vi "Tractor.vi"(1 "Y":dbl, 2 "X":dbl) -> (0 "XY Graph":cluster{dbl[], dbl[]}(graph))   [LabVIEW 2022 SP3]
panel:
  out "Array":dbl[](array[numeric])
  out "appended array":dbl[](array[numeric])
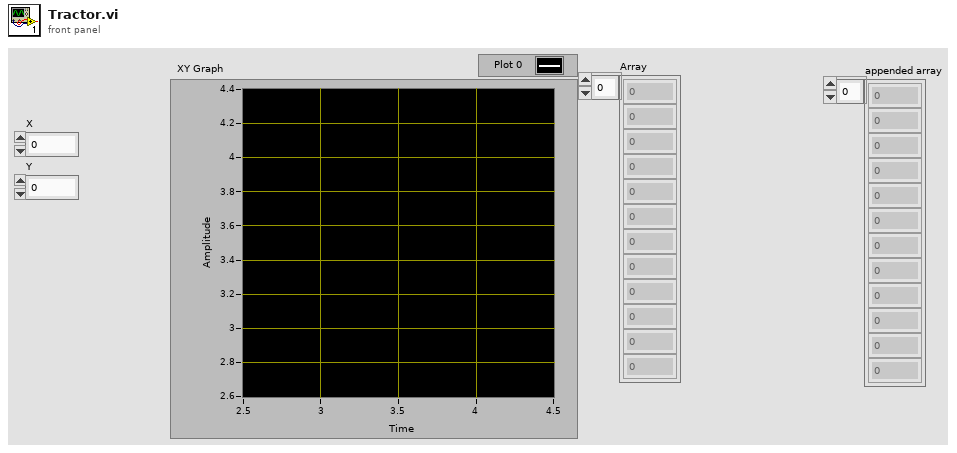
[diagram p1: front panel]
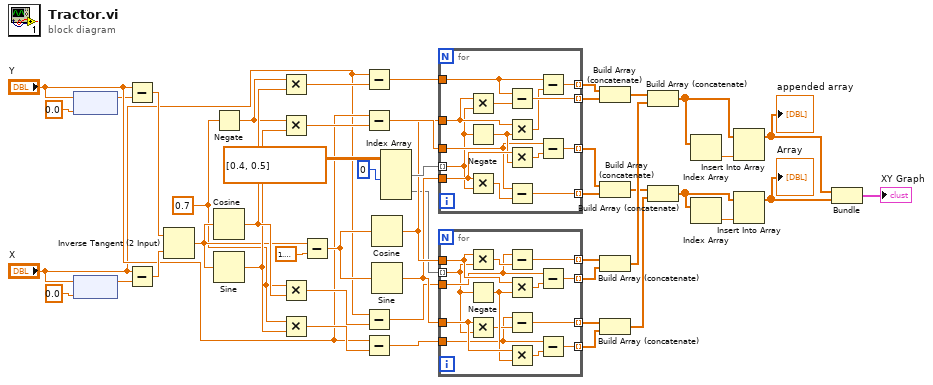
[diagram p0: block diagram]
diagram:
  w2 = 0.7 ("x")
  n1 = feedback #1(0.0 ("Y")) -> (w6:dbl)
  n2 = feedback-in #1("Y") -> ()
  n3 = feedback #2(0.0 ("Y")) -> (w3:dbl)
  n4 = feedback-in #2("X") -> ()
  n5 = Subtract(x="Y", y=w6) -> (x-y=w48:dbl)
  n6 = Subtract(x="X", y=w3) -> (x-y=w47:dbl)
  n7 = Inverse Tangent (2 Input)(1:w47, 2:w48) -> (0:w12:dbl)
  n8 = Negate(x=w2) -> (-x=w1:dbl)
  n9 = Cosine(x=w12) -> (cos(x)=w30:dbl)
  n10 = Sine(x=w12) -> (sin(x)=w29:dbl)
  n11 = Multiply(x=w1, y=w30) -> (x*y=w31:dbl)
  n12 = Multiply(x=w1, y=w29) -> (x*y=w44:dbl)
  n13 = Multiply(x=w2, y=w30) -> (x*y=w27:dbl)
  n14 = Multiply(x=w2, y=w29) -> (x*y=w26:dbl)
  n15 = Subtract(x=w12, y=1.5707963267948966) -> (x-y=w39:dbl)
  n16 = Subtract(x="X", y=w31) -> (x-y=w32:dbl)
  n17 = Subtract(x="Y", y=w44) -> (x-y=w36:dbl)
  n18 = Subtract(x="X", y=w27) -> (x-y=w28:dbl)
  n19 = Subtract(x="Y", y=w26) -> (x-y=w25:dbl)
  n20 = Cosine(x=w39) -> (cos(x)=w35:dbl)
  n21 = Sine(x=w39) -> (sin(x)=w34:dbl)
  n22 = Index Array(array=dbl[][] [[0.4, 0.5]] ("Figur array"), index (col) #1=0 ("disabled index (col)")) -> (element #1=w37:dbl[], element #2=w33:dbl[])  [unwired: 3 in]
  n23 = for {
    tunnel: w34 -> [w62]
    tunnel: w35 -> [w61]
    tunnel: [w59] -> w40 mode=indexing
    tunnel: [w58] -> w41 mode=indexing
    tunnel: [w57] -> w42 mode=indexing
    tunnel: [w56] -> w43 mode=indexing
    tunnel: w36 -> [w51]
    tunnel: w32 -> [w50]
    tunnel: w37 -> [w49] mode=indexing
    n24 = Multiply(x=w61, y=w49) -> (x*y=w55:dbl)
    n25 = Negate(x=w49) -> (-x=w60:dbl)
    n26 = Multiply(x=w62, y=w49) -> (x*y=w52:dbl)
    n27 = Subtract(x=w50, y=w55) -> (x-y=w58:dbl)
    n28 = Multiply(x=w61, y=w60) -> (x*y=w54:dbl)
    n29 = Multiply(x=w62, y=w60) -> (x*y=w53:dbl)
    n30 = Subtract(x=w51, y=w52) -> (x-y=w56:dbl)
    n31 = Subtract(x=w50, y=w54) -> (x-y=w59:dbl)
    n32 = Subtract(x=w51, y=w53) -> (x-y=w57:dbl)
  }
  n33 = for {
    tunnel: w34 -> [w76]
    tunnel: w35 -> [w75]
    tunnel: [w73] -> w18 mode=indexing
    tunnel: [w72] -> w17 mode=indexing
    tunnel: [w71] -> w20 mode=indexing
    tunnel: [w70] -> w19 mode=indexing
    tunnel: w25 -> [w65]
    tunnel: w28 -> [w64]
    tunnel: w33 -> [w63] mode=indexing
    n34 = Multiply(x=w75, y=w63) -> (x*y=w69:dbl)
    n35 = Negate(x=w63) -> (-x=w74:dbl)
    n36 = Multiply(x=w76, y=w63) -> (x*y=w66:dbl)
    n37 = Subtract(x=w64, y=w69) -> (x-y=w72:dbl)
    n38 = Multiply(x=w75, y=w74) -> (x*y=w68:dbl)
    n39 = Subtract(x=w65, y=w66) -> (x-y=w70:dbl)
    n40 = Multiply(x=w76, y=w74) -> (x*y=w67:dbl)
    n41 = Subtract(x=w64, y=w68) -> (x-y=w73:dbl)
    n42 = Subtract(x=w65, y=w67) -> (x-y=w71:dbl)
  }
  n43 = Build Array (concatenate)(w40, w41) -> (w24:dbl[])
  n44 = Build Array (concatenate)(w42, w43) -> (w22:dbl[])
  n45 = Build Array (concatenate)(w17, w18) -> (w23:dbl[])
  n46 = Build Array (concatenate)(w19, w20) -> (w21:dbl[])
  n47 = Build Array (concatenate)(w24, w23) -> (w16:dbl[])
  n48 = Build Array (concatenate)(w22, w21) -> (w14:dbl[])
  n49 = Index Array(array=w16) -> (element=w15:dbl)  [unwired: 1 in]
  n50 = Index Array(array=w14) -> (element=w13:dbl)  [unwired: 1 in]
  n51 = Insert Into Array(array=w16, new element=w15) -> (w10:dbl[])  [unwired: 1 in]
  "appended array" <- w10
  n52 = Insert Into Array(array=w14, new element=w13) -> (w9:dbl[])  [unwired: 1 in]
  "Array" <- w9
  n53 = Bundle(w10, w9) -> (→"XY Graph":cluster{dbl[], dbl[]})  [unwired: 1 in]
